vi "Untitled 1.vi"() -> ()   [LabVIEW 2019]
uses:
  Generated_client/RPC Messages/Greeter_req.ctl
  Generated_client/RPC Messages/Greeter_req_req_oneof/Greeter_req_req_oneof.lvclass
  Generated_client/RPC Messages/Greeter_MessageA.ctl
  Generated_client/RPC Messages/Greeter_req_req_oneof/Greeter_req_req_oneof.lvclass/Greeter_req_req_oneof.ctl
  Generated_client/RPC Messages/Greeter_res_res_oneof/Greeter_res_res_oneof.lvclass/Greeter_res_res_oneof.ctl
  Generated_client/Generated_client.lvlib
  Generated_client/RPC Messages/Greeter_res_res_oneof/Greeter_res_res_oneof.lvclass
panel:
  out "Get_Val":i32
  out "message_a":T1
  out "res_latitude":i32
  in  "Set_Val":string
  out "error out":errorcluster
  in  "Request Data":T2
  in  "address":string
  in  "error in":errorcluster
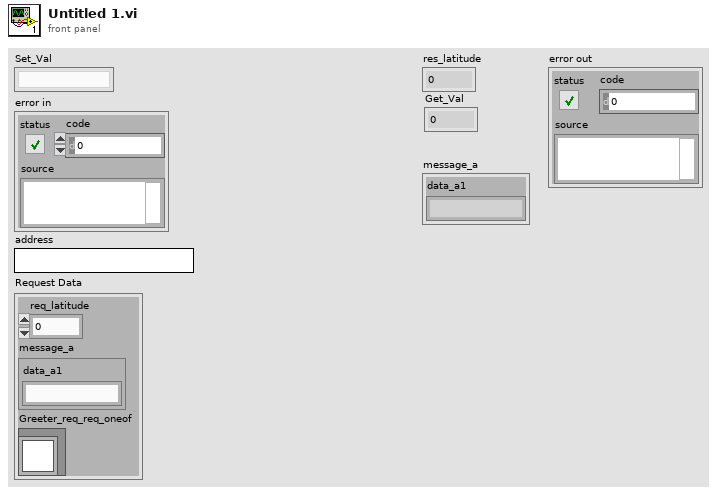
[diagram p1: front panel]
types:
  T1 = typedef "Generated_client.lvlib/Greeter_MessageA.ctl" = cluster{"data_a1":string}
  T2 = typedef "Generated_client.lvlib/Greeter_req.ctl" = cluster{"req_latitude":i32, "message_a":T1, "Greeter_req_req_oneof":refnum<class "Greeter_req_req_oneof.lvclass">}
  T3 = typedef "grpc-lvsupport-release.lvlib/grpcId.ctl" = u64
  T4 = typedef "Generated_client.lvlib/Greeter_res.ctl" = cluster{"res_latitude":i32, "Greeter_res_res_oneof":refnum<class "Greeter_res_res_oneof.lvclass">, "message_a":T1}
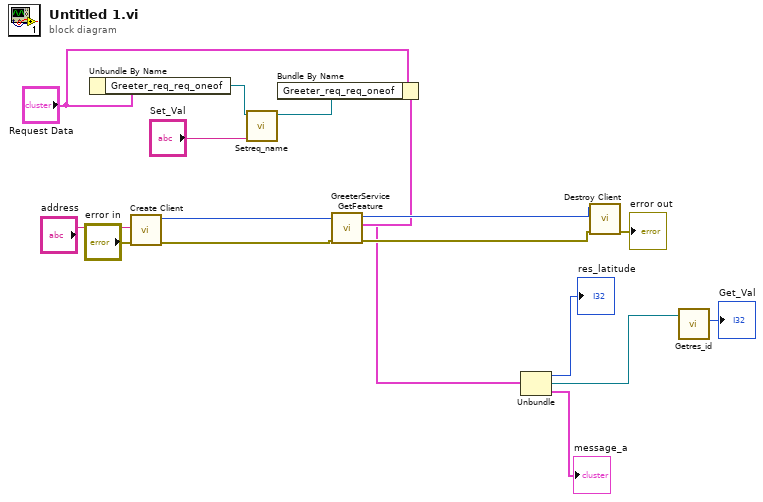
[diagram p0: block diagram]
diagram:
  n1 = Unbundle By Name("Request Data") -> ("Greeter_req_req_oneof"=w10:refnum<class "Greeter_req_req_oneof.lvclass">)
  n2 = call "Create Client.vi"("error in"="error in", "address"="address") -> ("error out"=w15:errorcluster, "gRPC ID Out"=w17:T3)  [unwired: 8 in]
  n3 = call "Setreq_name.vi"("Set_Val"="Set_Val", "OneOfTemplate in"=w10) -> ("OneOfTemplate out"=w8:refnum<class "Greeter_req_req_oneof.lvclass">)  [unwired: 8 in, 1 out]
  n4 = Bundle By Name(cluster="Request Data", "Greeter_req_req_oneof"=w8) -> (w7:T2)
  n5 = call "GreeterService GetFeature.vi"("error in"=w15, "Request Data"=w7, "gRPC ID"=w17) -> ("error out"=w14:errorcluster, "Response Data"=w5:T4, "gRPC ID out"=w16:T3)  [unwired: 6 in]
  n6 = Unbundle(w5) -> ("res_latitude"=→"res_latitude":i32, "Greeter_res_res_oneof"=w2:refnum<class "Greeter_res_res_oneof.lvclass">, "message_a"=→"message_a":T1)
  n7 = call "Destroy Client.vi"("error in"=w14, "gRPC ID"=w16) -> ("error out"=→"error out":errorcluster)  [unwired: 9 in]
  n8 = call "Getres_id.vi"("OneOfTemplate in"=w2) -> ("Get_Val"=→"Get_Val":i32)  [unwired: 8 in, 2 out]
